vi "Generate Sine Sweep.vi"() -> ()   [LabVIEW 2018]
uses:
  <vilib>/sound2/lvsound2.llb/Sound Data Format.ctl
  <vilib>/sound2/lvsound2.llb/Sampling Mode.ctl
  <vilib>/sound2/lvsound2.llb/Sound Input Read (DBL).vi
  <vilib>/sound2/lvsound2.llb/Sound Output Set Volume (Single).vi
  <vilib>/sound2/lvsound2.llb/Sound Output Write (DBL Single).vi
  <vilib>/addons/_NISVFA/_Generation/SoundVib_Generation.lvlib
panel:
  in  "amplitude":dbl=1.0 min=0.0 max=1.0 format="%.2f"
  out "Mic":waveform(dbl)[](graph)
  out "Done":bool
  in  "device In":u32
  out "Dur(s)":dbl
  out "size(s)":i32
  out "error out":errorcluster
  out "sound format":T1={"sample rate (S/s)"=51200.0, "number of channels"=1, "bits per sample"=16}
  in  "device Out":u32
  in  "chirp duration [s]":dbl=3.0
  in  "sampling info":cluster{"Fs":dbl, "#s":u32}={"Fs"=51200.0, "#s"=153600} {"Fs" format="%.2p"}
  in  "frequency spacing":enum16{"Linear", "Logarithmic"}(ring)=enum."Logarithmic"
  out "Waveform Graph":waveform(dbl)(graph)
  in  "frequency range [Hz]":cluster{"start":dbl, "stop":dbl}={"start"=20.0, "stop"=20000.0} {"stop" format="%.2f"; "start" format="%.2f"}
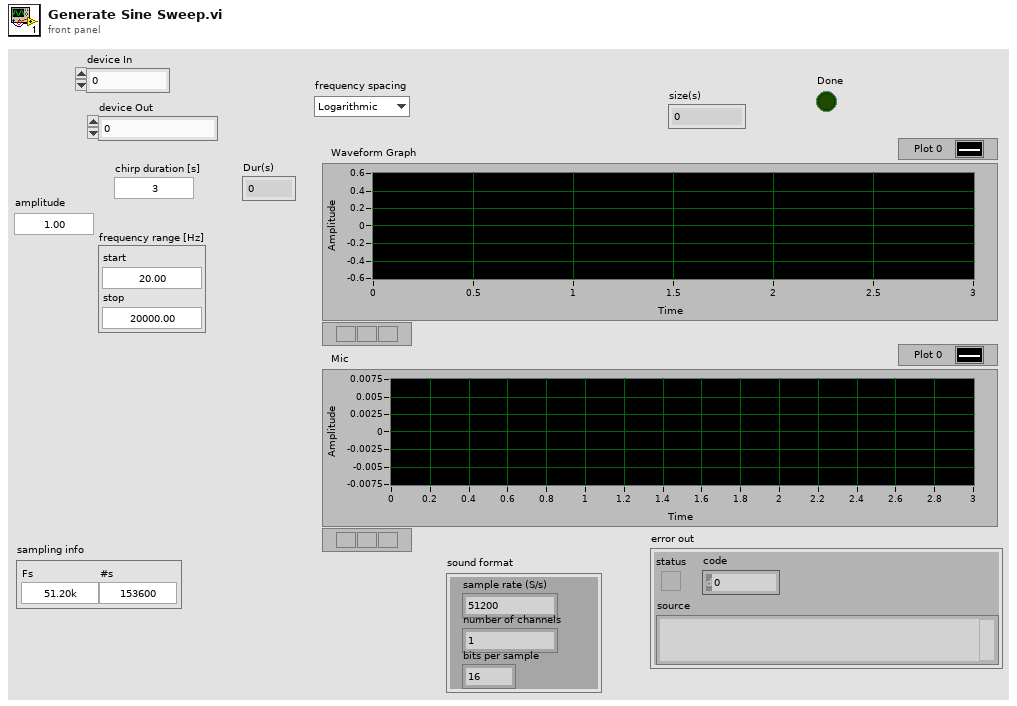
[diagram p1: front panel]
types:
  T1 = typedef "Sound Data Format.ctl" = cluster{"sample rate (S/s)":dbl, "number of channels":i32, "bits per sample":i32}
  T2 = typedef "Sampling Mode.ctl" = i32
  T3 = typedef "Sound Output Task ID.ctl" = u32
  T4 = typedef "Sound Input Task ID.ctl" = u32
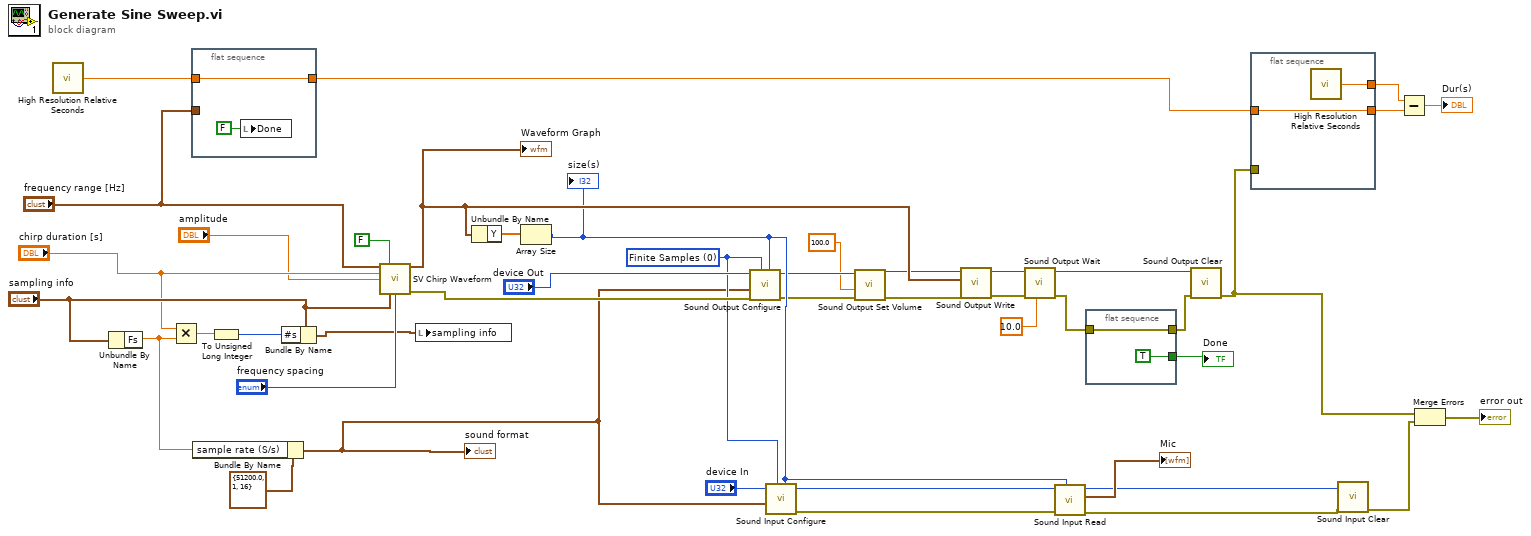
[diagram p0: block diagram]
diagram:
  w12 = T2 0 items=["Finite Samples", "Continuous Samples"] ("sample mode")
  n1 = call <vilib>:"High Resolution Relative Seconds.vi"() -> ("relative seconds"=w28:dbl)
  n2 = Unbundle By Name("sampling info") -> ("Fs"=w35:dbl)
  n3 = Multiply(x="chirp duration [s]", y=w35) -> (x*y=w38:dbl)
  n4 = flat-sequence {
    tunnel: w28 -> [w46]
    tunnel: "frequency range [Hz]" -> [_]
    tunnel: [w46] -> w26
    frame #0 {
      n5 = local write "Done"(FALSE ("Done")) -> ()
    }
  }
  n6 = Bundle By Name(cluster=T1 {"sample rate (S/s)"=51200.0, "number of channels"=1, "bits per sample"=16} ("sound format"), "sample rate (S/s)"=w35) -> (w5:T1)
  "sound format" <- w5
  n7 = To Unsigned Long Integer(number=w38) -> (unsigned 32bit integer=w37:u32)
  n8 = Bundle By Name(cluster="sampling info", "#s"=w37) -> (w36:cluster{"Fs":dbl, "#s":u32})
  n9 = call <vilib>:"SV Chirp Waveform.vi"("frequency range"="frequency range [Hz]", "reset signal (F)"=FALSE, "chirp duration [s]"="chirp duration [s]", "amplitude"="amplitude", "sampling info"="sampling info", "frequency spacing"="frequency spacing") -> ("chirp signal"=w41:waveform(dbl), "error out"=w43:errorcluster)  [unwired: 7 in, 1 out]
  "Waveform Graph" <- w41
  n10 = local write "sampling info"(w36) -> ()
  n11 = Unbundle By Name(w41) -> ("Y"=w40:dbl[])
  n12 = Array Size(array=w40) -> (size(s)=w19:i32)
  "size(s)" <- w19
  n13 = call <vilib>:"Sound Output Configure.vi"("number of samples/ch"=w19, "sample mode"=w12, "error in (no error)"=w43, "sound format"=w5, "device ID"="device Out") -> ("error out"=w10:errorcluster, "task ID"=w11:T3)  [unwired: 5 in]
  n14 = call <vilib>:"Sound Input Configure.vi"("number of samples/ch"=w19, "sample mode"=w12, "sound format"=w5, "device ID"="device In") -> ("error out"=w20:errorcluster, "task ID"=w21:T4)  [unwired: 6 in]
  n15 = call-poly <vilib>:"Sound Output Set Volume.vi"("error in (no error)"=w10, "volume"=100.0, "task ID"=w11) -> ("error out"=w9:errorcluster, "task ID out"=w8:T3)  [unwired: 7 in]
  n16 = call-poly <vilib>:"Sound Output Write.vi"("error in (no error)"=w9, "data"=w41, "task ID"=w8) -> ("error out"=w31:errorcluster, "task ID out"=w32:T3)  [unwired: 7 in]
  n17 = call <vilib>:"Sound Output Wait.vi"("timeout (sec)"=10.0, "error in (no error)"=w31, "task ID"=w32) -> ("error out"=w18:errorcluster, "task ID out"=w30:T3)  [unwired: 7 in]
  n18 = call-poly <vilib>:"Sound Input Read.vi"("number of samples/ch"=w19, "error in (no error)"=w20, "task ID"=w21) -> ("error out"=w1:errorcluster, "data"=→"Mic":waveform(dbl)[], "task ID out"=w2:T4)  [unwired: 6 in]
  n19 = flat-sequence {
    tunnel: w18 -> [w48]
    tunnel: [w48] -> w17
    tunnel: [TRUE] -> w16
    frame #0 {
    }
  }
  n20 = call <vilib>:"Sound Output Clear.vi"("error in (no error)"=w17, "task ID"=w30) -> ("error out"=w15:errorcluster)  [unwired: 9 in]
  n21 = flat-sequence {
    tunnel: w26 -> [w50]
    tunnel: [w50] -> w25
    tunnel: w15 -> [_]
    tunnel: [w49] -> w24
    frame #0 {
      n22 = call <vilib>:"High Resolution Relative Seconds.vi"() -> ("relative seconds"=w49:dbl)
    }
  }
  n23 = call <vilib>:"Sound Input Clear.vi"("error in (no error)"=w1, "task ID"=w2) -> ("error out"=w14:errorcluster)  [unwired: 9 in]
  n24 = Subtract(x=w24, y=w25) -> (x-y=→"Dur(s)":dbl)
  n25 = Merge Errors(w15, w14) -> (→"error out":errorcluster)
  "Done" <- w16
